vi "fft output to real signal.vi"() -> ()   [LabVIEW 2010]
uses:
  <vilib>/rvi/FXPMathLib/FxpInterpret/XNode/nifxpmath_Interpret.xnode
  <vilib>/Analysis/2dsp.llb/Inverse Real FFT.vi
  <vilib>/Analysis/NI_AALPro.lvlib
panel:
  out "Waveform Graph 3":dbl[](graph)
  in  "Log Mag":i32[](array[numeric])=array[10000 elements]
  in  "Im1 3":i16[](array[numeric])=array[10000 elements]
  in  "Re1 3":i16[](array[numeric])=array[10000 elements]
  out "Waveform Graph 2":dbl[](graph)
  out "Waveform Graph":dbl[](graph)=[0.0013443231582641602, 0.009328283740266213, 0.01665657369087733, 0.0074937709819613875, 0.014597284621130222, -0.00020039519176043188, 0.02212248617670058, 0.019572909166947785, -5.522809960701799e-06, 0.0030579312385367718, -0.0011017547396133538, 0.012496666409438644, 0.0033977673822338248, 0.009327941888197203, 0.00790739093659378, 0.00324635276992021, 0.012784517380908304, 0.01678925480080535, -0.0024760847108160206, -0.013601985803444919, 0.0190453068721778, 0.0002259143606861808, 0.008123668724325045, 0.00021194432114504235, 0.007220344483716528, 0.0015953701316602812, 0.008026984740082968, 0.003165249077891774, 0.013837141554459817, -0.0018901896972592514, 0.004009335080789208, -0.015981262048713623, -0.003055080665293577, 0.006757276215648919, 0.011143635287443578, 0.007982287567807734, 0.010984855900208437, 0.0007804848128102593, 0.012865857714949108, 0.026133471272553273, 0.0005232584668258882, 0.005834532957324823, -0.004884000036303867, 0.011474035954591176, 0.0022973366849122056, 0.007676746741121305, 0.007526365506647573, 0.0023302984243481605, 0.008996638243063064, 0.018725772099461153, 0.004004449098521394, -0.016956718452396723, 0.013888371987740414, 0.002795702196854375, 0.005023119724665563, 0.0014828367858530566, 0.0038201100198896596, 0.002005340304001158, 0.00469804203489217, 0.0028165872194784647, 0.011718281018712378, 0.00199113356669734, 0.003009721007275916, -0.012271685413787295, -0.012901710835042619, 0.0032799754834772835, 0.0040366701681482636, 0.007361039503742175, 0.005790797915210081, 0.0017055867197399604, 0.0017600841940617331, 0.028788741575559988, 0.0010935062357852019, 0.007928902533717707, -0.007763381570267349, 0.008919609655347053, 0.0009789350442093083, 0.004947361555411334, 0.006182979565066396, 0.001233193256757842, 0.004039837731759147, 0.01794986796139517, 0.009998656885496164, -0.017522171703696295, 0.006770440377944936, 0.00512623084522261, 0.0013667105982569593, 0.002676577996641972, 2.8097050724767633e-05, 0.0023106042611368127, 0.0008260297265834295, 0.0022356346592576257, 0.007946569613381886, 0.005706989102484808, 0.001713078198844054, -0.006501318919181848, -0.020701846574672295, -0.0004756356821032483, -0.0034853872870562524, 0.00582723424924648, -4.612480299289357e-05, 0.0025745705612483663, -0.009346777376794176, 0.027331182979049545, 0.0017136568513873044, 0.008961911421860942, -0.009237486770530039, 0.005136089894557029, -0.000229783661362309, 0.0017674856175168932, 0.0040828951773568805, 0.00016684537878847334, -0.0012861650309019803, 0.014704926312474668, 0.014760127543856498, -0.015198694010095774, -0.0011157986651634648, 0.0069162554657452, -0.002254460569622385, 0.003710349250102243, -0.003446078538563074, 0.002535895567668497, -0.0028811042898947373, 0.0016247000946398795, 0.0032734973548561187, 0.00885764636422768, 0.000457790958252712, 0.0005599935669895651, -0.025050759315490723, -0.003917036299966406, -0.010203821425034839, 0.0037109133265186985, -0.005576327119715211, 0.0033958647240763884, -0.0187888964086819, 0.02193970242413782, 0.0023808138438635162, 0.008984548590052264, -0.009049308894950987, 0.0009226385004196284, -0.0011206179818098138, -0.0014520808493189187, 0.0017218617709807826, -0.0006034557439638811, -0.006142739181829694, 0.009528540549875304, 0.017541986493847264, -0.010262714099435785, -0.008540605949627253, 0.007966832654043028, -0.005235018873054959, 0.0044800045798794605, -0.006194580416717728, 0.0026660653853135333, -0.005859596441216282, 0.0009773863225038786, -0.001638086185165116, 0.010943058096095552, -0.0005985184583909248, 0.0077853645348875886, -0.02529400585598377, -0.006431298994949641, -0.01509651869223753, 0.0012786447178075768, -0.009974776446671482, 0.003929166148753089, -0.025062360328309136, 0.013531860847676734, 0.0029668339204212547, 0.00791346377301647, -0.007138361748568264, -0.0031844625965817175, -0.0016046387239466119, -0.0041380134045758505, -0.0006846836155743833, -0.001032727219959148, -0.009765885283871137, 0.0031618937199808287, 0.017956690235909664, -0.0034900416409245497, -0.014425535875160253, 0.008058067047010571, -0.007131934917535764, 0.004923706188454897, -0.007641364677097374, 0.0026467292121099533, -0.007680335688533465, 0.0004875428301553924, -0.00601719512485266, 0.011654550958823779, -0.0012861336706713493, 0.01413305145947654, -0.021334326705337126, -0.007731793083146804, -0.017357321409410154, -0.001031266258789016, -0.012605199869064951, 0.004162769697106895, -0.02722120169640587, 0.0033526167899944797, 0.0033765401000995228, 0.005841154173995276, -0.003905200235458285, -0.006504664978656117, -0.001518528111415395, -0.005970556903962497, -0.0026977649441710444, -0.0010255062085794287, -0.011651255370488398, -0.0034129671805393576, 0.015849412096512708, 0.004072532748335549, -0.01783024506652309, 0.007195510878588977, -0.007742818236824435, 0.004726785280682453, -0.007745193850917978, 0.0025044741475733386, -0.008091517504780366, 0.00017729957257255524, -0.009222522847255195, 0.01077533954235207, -0.001535242218697148, 0.0185009042416472, -0.014028832411226898, -0.007629160930707667, -0.01680948723777248, -0.0030094114649847066, -0.013131227499428607, 0.003936123195551828, -0.025104555682492074, -0.007177990980371357, 0.0034542051915313937, 0.0031587721868950357, 8.988130163316375e-05, -0.008681083063503892, -0.0010511454090181213, -0.00667825618933762, -0.004143724859573905, -0.0007083179864898507, -0.011606836059039694, -0.00935038655985125, 0.011532409345090804, 0.011131055470081919, -0.018351561273097276, 0.005345585725920276, -0.006993764990180353, 0.004018582622529068, -0.0065245179793835106, 0.0020473648280574215, -0.007165637909829765, -7.261213250412085e-05, -0.010953040001153817, 0.008425921937179112, -0.0014740005060327232, 0.02021576321653155, -0.004425168037414551, -0.006242862427408904, -0.013608010108093357, -0.004405727551962653, -0.011518687494293797, 0.003249572660805981, -0.01906713281863228, -0.016520949828005057, 0.003057253238478082, -1.2424337115606726e-05, 0.004157297386622619, -0.009450388976214225, -0.00038161723897024366, -0.0063058908079131675, -0.00488934957871016, -0.00018908362158703146, -0.009762044651310723, -0.01377212532084288, 0.005456592081952302, 0.01655072578422172, -0.016077866166163638, 0.002737279422836127, -0.0051605046927350835, 0.0027217490955840397, -0.004254968772618764, 0.0013626156295019121, -0.005099123615935151, -0.0002640267456396751, -0.010946663144537403, 0.004783233597200119, -0.0011484277271569098, 0.01882387927848595, 0.005879303798834477, -0.00391530363825277, -0.008331316451183938, -0.00516101598534263, -0.008188069675446023, 0.001991448621110211, -0.0100877500027917, -0.023392010454496254, 0.002201399462122841, -0.0031526359617420436, 0.0075775490652922935, -0.008842886866119098, 0.00036428397174266547, -0.005057470370927577, -0.004920414189049586, 0.0002765271605560658, -0.006439015710754456, -0.01615971764925691, -0.0014670442366619225, 0.01942763803947864, -0.011446323333518322, -0.00035569379766564515, -0.0026074925879710385, 0.000942719479967154, -0.0014430621199655502, 0.00033948755741241513, -0.0023753109353251405, -0.0005024618089753247, -0.009405101386868309, 0.0002983860821903189, -0.0007602952092062559, 0.014466389326686034, 0.015094923344197892, -0.0011208438714745746, -0.0018914578301480215, -0.005251534868137923, -0.003710872772153908, 0.000334282618940545, 0.0002159254248882683, -0.026798711079322836, 0.0008638100475162609, -0.005988476358256805, 0.009682938303843381, -0.007024985399149673, 0.0008541659585674056, -0.0031363167715065176, -0.004404216133365706, 0.0005067801578918477, -0.0023312106221884234, -0.016270333933748164, -0.00834985692963138, 0.019168477635313364, -0.00518623098067836, -0.00357056240209283, 0.0001496846069047415, -0.0011857117434227842, 0.001434530087788224, -0.0008786660216772444, 0.0005477968521902469, -0.0008573415076385681, -0.006641958723514534, -0.004418810825394484, -0.0004550869960044581, 0.0077179716720554925, 0.02191470310249745, 0.001642803640854073, 0.004608935285649953, -0.0047693894932437, 0.0010855325272105686, -0.0015992387414586744, 0.01033175405207362, -0.026381442025083975, -0.0008413766143849518, -0.00809861714874147, 0.010062684865409663, -0.004343449233627236, 0.0010063977720642138, -0.001036085236925854, -0.0033895284997637037, 0.0004862570757197598, 0.0018918160507565918, -0.014159590128952444, -0.014241681098492555, 0.015702493421212726, 0.001560197157064691, -0.006525831626103761, 0.002648128701190297, -0.0033742036589996306, 0.003782343777147568, -0.0022315161300231635, 0.003098652057317958, -0.0014228201878899807, -0.0030832188951940218, -0.008731889559954291, -0.00037708856356387117, -0.0005003026517018312, 0.02502119541168213, 0.00387054745083019, 0.010120485114400543, -0.003800710392889648, 0.005461148199217978, -0.003576282446597871, 0.01858039100897846, -0.022219745879284228, -0.002702689350509943, -0.009310741790339562, 0.00867507085326919, -0.0013148817933901847, 0.0006980336749396043, 0.0009611770774033655, -0.002235105123269453, 1.891352066847249e-05, 0.005558095148486014, -0.010138522959877697, -0.018205163745713494, 0.009566598825814964, 0.007841049712294504, -0.00876148962843517, 0.004418384197798583, -0.005339047835921855, 0.005309023498727438, -0.00358715679557395, 0.004886859930152269, -0.0019817690869566532, 0.0006322521353685842, -0.012005844972778233, -0.0004956945050212484, -0.008939830120240196, 0.024116301429718257, 0.00524677693955296, 0.013835740809470863, -0.0025827120867554926, 0.008678408279546407, -0.005235970491650085, 0.02367763616462347, -0.014961556036130643, -0.004404326122841595, -0.009375488753440898, 0.005639899137479056, 0.0016509463710425126, 6.19837535139299e-06, 0.002527780884083693, -0.0009436443557822721, -0.0006555648594904033, 0.008051268666044952, -0.004927238428734618, -0.01973293476151957, 0.0017179721033994816, 0.012589846293546605, -0.009923860872285348, 0.005271314886009451, -0.006820663014053424, 0.005732907242004762, -0.004631050604619998, 0.00566288160937124, -0.0025315151440263306, 0.003983769048819232, -0.013735764806072859, -0.0008460781991056153, -0.01626558202438018, 0.01917115493714865, 0.005537890288432842, 0.015122743991274043, -0.0012245845967285053, 0.01033028033316248, -0.00644839882429928, 0.024911006291575236, -0.005702939001754688, -0.0057159942010358775, -0.00827413377219043, 0.0014936879614611343, 0.004068951838361099, -0.0009244633122924405, 0.003460749477555096, 0.00019665678974167692, -0.0015135506682150968, 0.009126045902554388, 0.0008441306366969003, -0.0184414736449078, -0.0066552880679562314, 0.015202902824488532, -0.009838911968815091, 0.00506001119876975, -0.007450764939717033, 0.0050618471911703196, -0.0052213667445563, 0.005383613341273282, -0.0029218475004441575, 0.006480661214094567, -0.013582043773893266, -0.0012788898013643551, -0.021302869726682806, 0.011199974754251356, 0.004758405017250147, 0.013947074040122198, 0.00014685514351092427, 0.010260284246957503, -0.0068255577211612595, 0.022172465991600068, 0.004276243267082424, -0.006370639499532573, -0.006091710792131358, -0.0030539197653544443, 0.005713539561115033, -0.0019101840606338735, 0.0036814703866895303, 0.001121277850298582, -0.002320361880706454, 0.008588431199897967, 0.0063323417276165, -0.014522148752521618, -0.014174120875670389, 0.015343915419531753, -0.00839304937984395, 0.00393895486315794, -0.0070735636821383525, 0.003460569107610339, -0.005117402255037688, 0.004102163929189799, -0.0029672281076098617, 0.007895550420292281, -0.011485837633858537, -0.0016021896196202036, -0.02327802268006435]
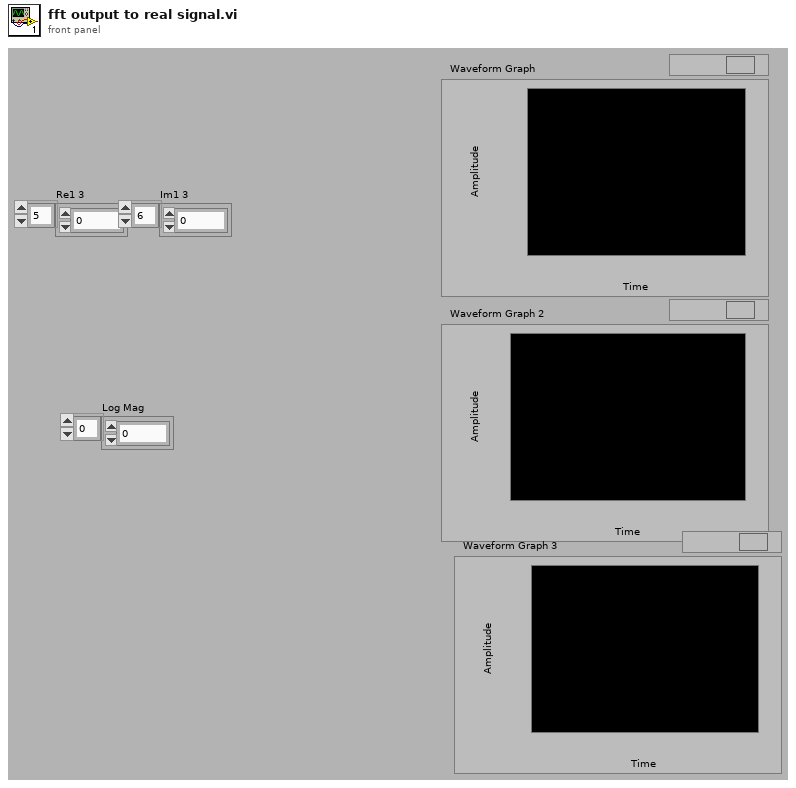
[diagram p1: front panel]
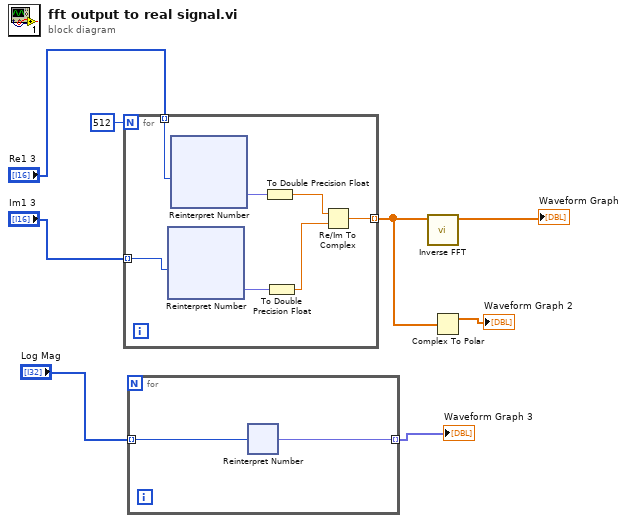
[diagram p0: block diagram]
diagram:
  n1 = for {
    N: 512 -> [_]
    tunnel: "Re1 3" -> [w15] mode=indexing
    tunnel: "Im1 3" -> [w14] mode=indexing
    tunnel: [w9] -> w6 mode=indexing
    n2 = xnode "Reinterpret Number"("x"=w14) -> ("y"=w12:fxp<+/-,16,1>)
    n3 = xnode "Reinterpret Number"("x"=w15) -> ("y"=w13:fxp<+/-,16,1>)
    n4 = To Double Precision Float(number=w13) -> (double precision float=w11:dbl)
    n5 = To Double Precision Float(number=w12) -> (double precision float=w10:dbl)
    n6 = Re/Im To Complex(1:w10, 2:w11) -> (0:w9:cdb)
  }
  n7 = for {
    tunnel: "Log Mag" -> [w21] mode=indexing
    tunnel: [w20] -> w1 mode=indexing
    n8 = xnode "Reinterpret Number"("x"=w21) -> ("y"=w20:fxp<+/-,32,16>)
  }
  "Waveform Graph 3" <- w1
  n9 = call-poly <vilib>:"Inverse FFT.vi"("FFT {X}"=w6) -> ("X"=→"Waveform Graph":dbl[])  [unwired: 9 in, 1 out]
  n10 = Complex To Polar(r * e^(i*theta)=w6) -> (r=→"Waveform Graph 2":dbl[])  [unwired: 1 out]
